vi "Parse.vi"(8 "Error In":errorcluster, 11 "object in":refnum<class "2021_17.lvclass">) -> (0 "Error Out":errorcluster, 3 "object out":refnum<class "2021_17.lvclass">)   [LabVIEW 2020, in "2021_17.lvclass"]
uses:
  2021_17.lvclass
  2021_17.lvclass/2021_17.ctl
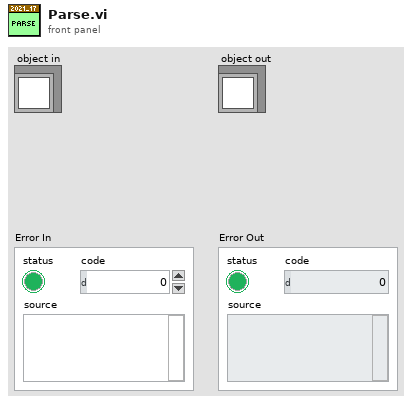
[diagram p1: front panel]
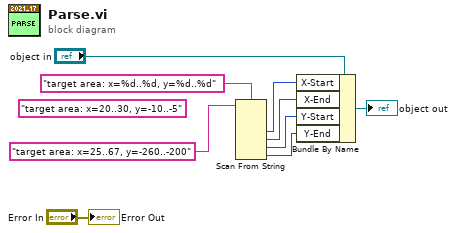
[diagram p0: block diagram]
diagram:
  (unwired) "target area: x=20..30, y=-10..-5" ("PuzzleInput")
  n1 = Scan From String(format string="target area: x=%d..%d, y=%d..%d", input string="target area: x=25..67, y=-260..-200" ("PuzzleInput")) -> (output 1=w5:i32, output 2=w4:i32, output 3=w3:i32, output 4=w2:i32)  [unwired: 6 in, 3 out]
  n2 = Bundle By Name(cluster="object in", "X-Start"=w5, "X-End"=w4, "Y-Start"=w3, "Y-End"=w2) -> (→"object out":refnum<class "2021_17.lvclass">)
  "Error Out" <- "Error In"
